vi "FlpLib CalcSymDQ 2.vi"(0 "A":sgl, 1 "ak":sgl, 2 "bk":sgl, 5 "B":sgl, 7 "C":sgl, 9 "trigSignals":T1, 11 "State In":sgl[](array[numeric])=[0.0, 0.0, 0.0, 0.0, 0.0, 0.0, 0.0, 0.0, 0.0, 0.0, 0.0, 0.0], 12 "Speed":sgl format="%#_13g", 13 "SpeedThreshhold":sgl format="%#_13g") -> (4 "D1":sgl, 6 "Q1":sgl, 8 "D2":sgl, 10 "Q2":sgl, 15 "State Out":sgl[](array[numeric]))   [LabVIEW 2017]
uses:
  ABCtoAlphaBeta_3PhaseUnitaryMagnitude/FlpLib ABCtoAlphaBeta_3PhaseUnitaryMagnitude 2.vi
  AlphaBetaToDQ_noSine/FlpLib AlphaBetaToDQ_noSine 2.vi
  <userlib>/_NI FLP Library/FPGA/outsideSCTL/FlpLib Subtract Shared Instance 2.vi
  Filter/IIRDirectFormIITrans1stOrder/FlpLib IIRDirectFormIITrans1stOrder 2.vi
  <userlib>/_NI FLP Library/FPGA/outsideSCTL/FlpLib In Range and Coerce Shared Instance 2.vi
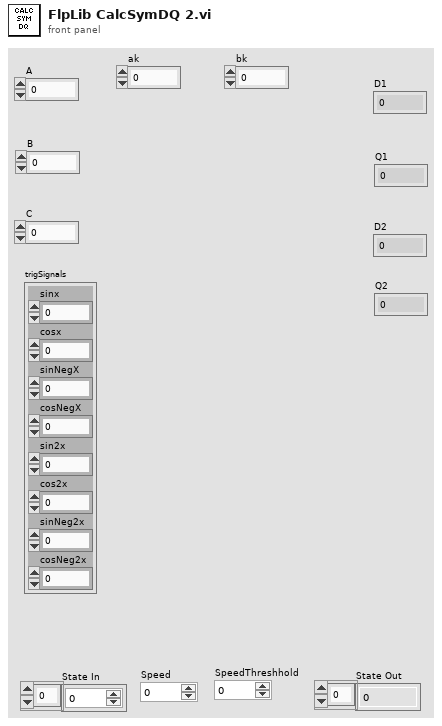
[diagram p1: front panel]
types:
  T1 = typedef "trigSignals" = cluster{"sinx":sgl, "cosx":sgl, "sinNegX":sgl, "cosNegX":sgl, "sin2x":sgl, "cos2x":sgl, "sinNeg2x":sgl, "cosNeg2x":sgl}
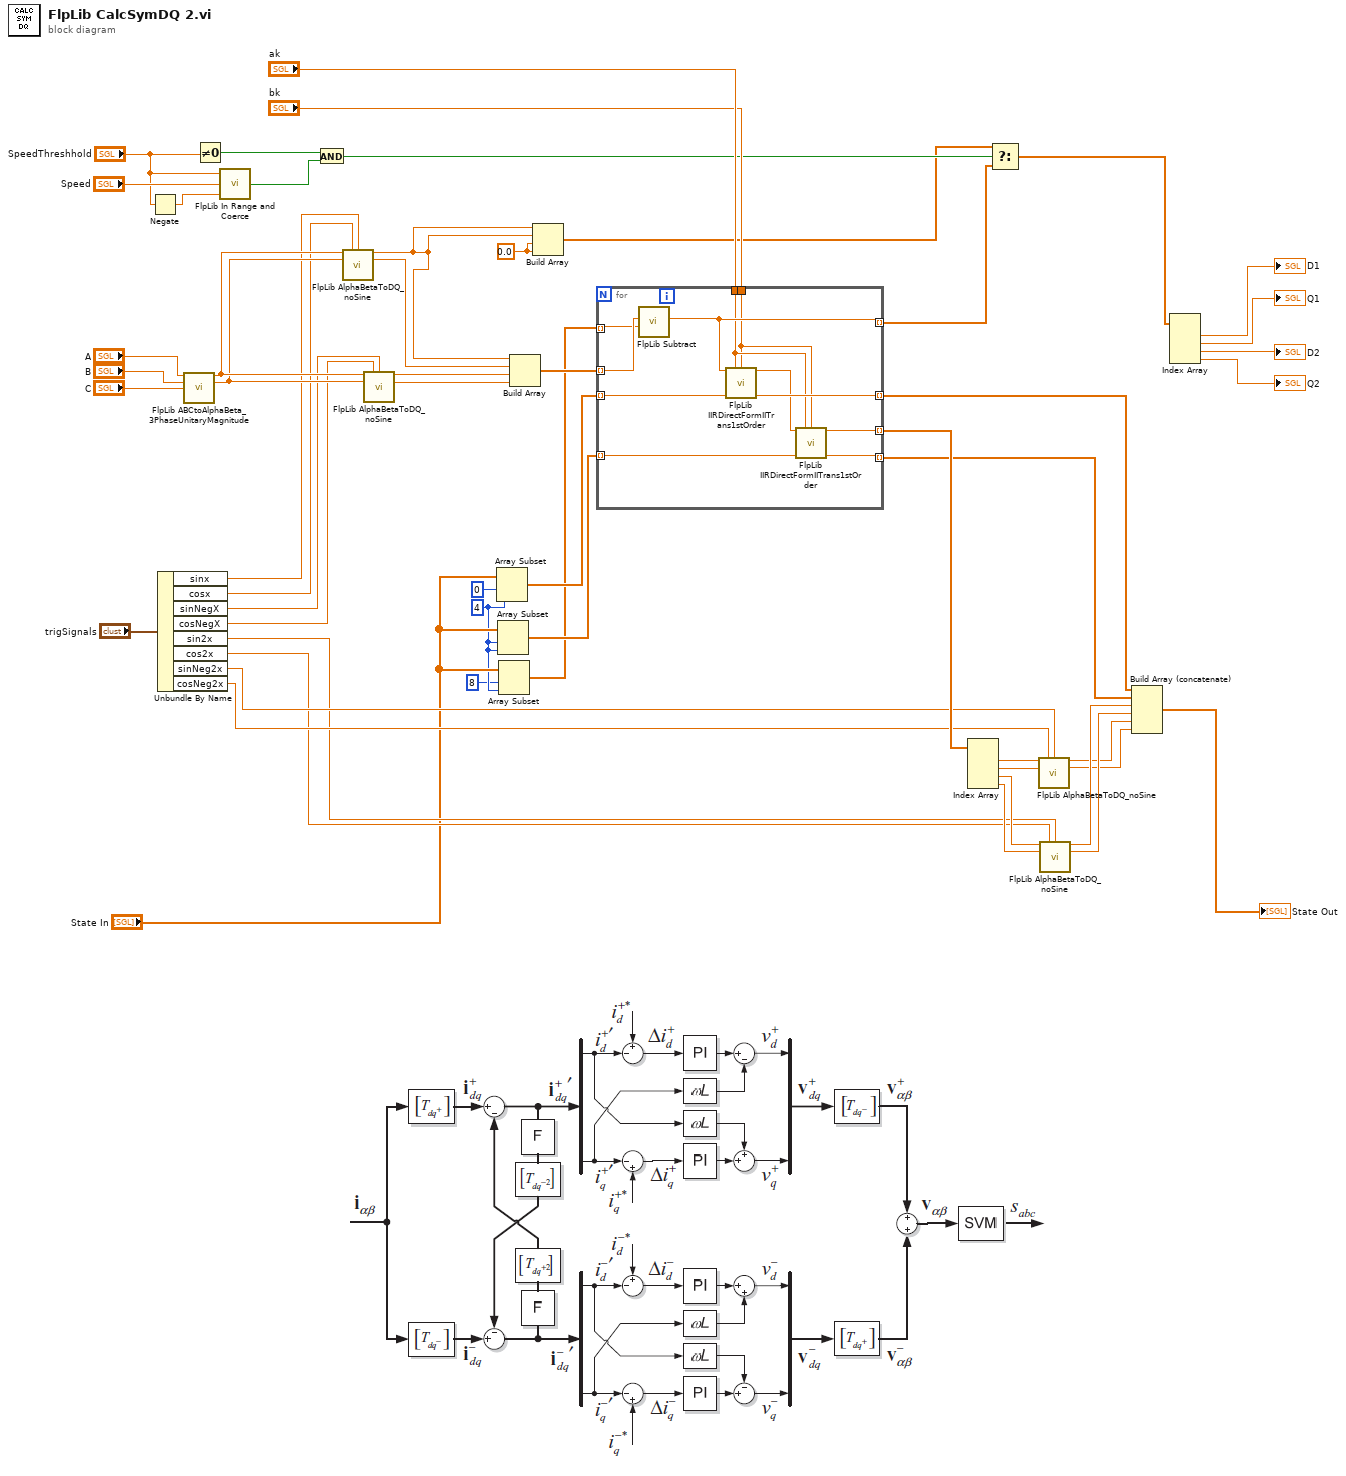
[diagram p0: block diagram]
diagram:
  w8 = sgl 0.0 ("element")
  w15 = 4 ("length")
  n1 = Negate(x="SpeedThreshhold") -> (-x=w10:sgl)
  n2 = Unbundle By Name("trigSignals") -> ("sinx"=w42:sgl, "cosx"=w41:sgl, "sinNegX"=w40:sgl, "cosNegX"=w39:sgl, "sin2x"=w29:sgl, "cos2x"=w28:sgl, "sinNeg2x"=w31:sgl, "cosNeg2x"=w30:sgl)
  n3 = call-poly "FlpLib ABCtoAlphaBeta_3PhaseUnitaryMagnitude.vi"("A"="A", "B"="B", "C"="C") -> ("alpha"=w45:sgl, "beta"=w44:sgl)  [unwired: 11 in]
  n4 = Not Equal To 0?(x="SpeedThreshhold") -> (x != 0?=w2:bool)
  n5 = call-poly <userlib>:"FlpLib In Range and Coerce.vi"("lower limit"=w10, "x"="Speed", "upper limit"="SpeedThreshhold") -> ("in range?"=w7:bool)  [unwired: 1 in, 1 out]
  n6 = And(x=w2, y=w7) -> (x .and. y?=w6:bool)
  n7 = call-poly "FlpLib AlphaBetaToDQ_noSine.vi"("alpha"=w45, "cosx"=w41, "sinx"=w42, "beta"=w44) -> ("direct"=w9:sgl, "quadrature"=w38:sgl)  [unwired: 10 in]
  n8 = call-poly "FlpLib AlphaBetaToDQ_noSine.vi"("alpha"=w45, "cosx"=w39, "sinx"=w40, "beta"=w44) -> ("direct"=w37:sgl, "quadrature"=w36:sgl)  [unwired: 10 in]
  n9 = Array Subset(array="State In", index=0, length=w15) -> (w20:sgl[])
  n10 = Array Subset(array="State In", index=w15, length=w15) -> (w13:sgl[])
  n11 = Array Subset(array="State In", index=8, length=w15) -> (w12:sgl[])
  n12 = Build Array(w9, w38, w37, w36) -> (w54:sgl[])
  n13 = Build Array(w9, w9, w8, w8) -> (w5:sgl[])
  n14 = for {
    tunnel: w54 -> [w63] mode=indexing
    tunnel: [w59] -> w53 mode=indexing
    tunnel: w20 -> [w65] mode=indexing
    tunnel: [w64] -> w19 mode=indexing
    tunnel: w12 -> [w62] mode=indexing
    tunnel: [w61] -> w4 mode=indexing
    tunnel: "ak" -> [w58]
    tunnel: "bk" -> [w57]
    tunnel: [w56] -> w17 mode=indexing
    tunnel: w13 -> [w55] mode=indexing
    n15 = call-poly <userlib>:"FlpLib Subtract.vi"("y"=w62, "x"=w63) -> ("x-y"=w61:sgl)  [unwired: 5 in]
    n16 = call-poly "FlpLib IIRDirectFormIITrans1stOrder.vi"("xn"=w61, "ak"=w58, "bk"=w57, "stateIn"=w65) -> ("yn"=w60:sgl, "stateOut"=w64:sgl)  [unwired: 10 in]
    n17 = call-poly "FlpLib IIRDirectFormIITrans1stOrder.vi"("xn"=w60, "ak"=w58, "bk"=w57, "stateIn"=w55) -> ("yn"=w59:sgl, "stateOut"=w56:sgl)  [unwired: 10 in]
  }
  n18 = Index Array(array=w53) -> (element #1=w52:sgl, element #2=w51:sgl, element #3=w50:sgl, element #4=w49:sgl)  [unwired: 4 in]
  n19 = Select(t=w5, s=w6, f=w4) -> (s? t:f=w3:sgl[])
  n20 = call-poly "FlpLib AlphaBetaToDQ_noSine.vi"("alpha"=w52, "cosx"=w30, "sinx"=w31, "beta"=w51) -> ("direct"=w25:sgl, "quadrature"=w24:sgl)  [unwired: 10 in]
  n21 = call-poly "FlpLib AlphaBetaToDQ_noSine.vi"("alpha"=w50, "cosx"=w28, "sinx"=w29, "beta"=w49) -> ("direct"=w27:sgl, "quadrature"=w26:sgl)  [unwired: 10 in]
  n22 = Build Array (concatenate)(w19, w17, w27, w26, w25, w24) -> (→"State Out":sgl[])
  n23 = Index Array(array=w3) -> (element #1=→"D1":sgl, element #2=→"Q1":sgl, element #3=→"D2":sgl, element #4=→"Q2":sgl)  [unwired: 4 in]
